vi "VI Scripting with Structures - Event Structure.vi"   [LabVIEW 2019]
doc: "This example contains sample code demonstrating common VI Scripting navigational tasks relating to Event Structures."
uses:
  <vilib>/Utility/traverseref.llb/TRef TravTarget.ctl
  <vilib>/event_ctls.llb/lveventtype.ctl
  <vilib>/Utility/traverseref.llb/VI Scripting - Traverse.lvlib
panel:
  # "Overview: Illustrates several EventStructure properties and methods used for inspecting and modifying Event Structures with VI Scripting.\nInstructions:\nOpen the block diagram of this VI to see several examples of properties and methods related to Event Structures and VI Scripting.\n\nNote: Browse the diagram of this example to learn about VI Scripting concepts. This example is not meant to be run."
types:
  T1 = typedef "lveventtype.ctl" = enum32{"Null", "Timeout", "Annotation Menu Selection", "Annotation Menu Selection?", "App Instance Close", "App Instance Close?", "Autoscale Range Change", "Bookmark Info Change", "Cell Edit", "Cell Edit?", "Cursor Grab", "Cursor Grab?", "Cursor Menu Selection", "Cursor Menu Selection?", "Cursor Move", "Cursor Release", "Data Change", "Direction Change", "Display State Change", "Drag Ended", "Drag Enter", "Drag Leave", "Drag Over", "Drag Source Update", "Drag Starting", "Drag Starting?", "Drop", "Exec State Change", "Key Down", "Key Down?", "Key Repeat", "Key Repeat?", "Key Up", "Listbox Double Click", "Menu Activation?", "Menu Selection (App)", "Menu Selection? (App)", "Menu Selection (User)", "Mouse Down", "Mouse Down?", "Mouse Enter", "Mouse Leave", "Mouse Move", "Mouse Up", "Mouse Wheel", "NI Security User Change (App)", "Pane Size", "Panel Close", "Panel Close?", "Panel Resize", "Plot Attribute Change", "Scale Range Change", "Shortcut Menu Activation?", "Shortcut Menu Selection (App)", "Shortcut Menu Selection? (App)", "Shortcut Menu Selection (User)", "Tree Double Click", "Tree Drag", "Tree Drag?", "Tree Drop", "Tree Drop?", "Tree Item Close", "Tree Item Close?", "Tree Item Open", "Tree Item Open?", "User Event", "Value Change"}
  T2 = cluster{"Event Type":T1, "Event Registration Index":i32}[]
  T3 = enum32{"Null", "Timeout", "Annotation Menu Selection", "Annotation Menu Selection?", "App Instance Close", "App Instance Close?", "Autoscale Range Change", "Bookmark Info Change", "Cell Edit", "Cell Edit?", "Cursor Grab", "Cursor Grab?", "Cursor Menu Selection", "Cursor Menu Selection?", "Cursor Move", "Cursor Release", "Data Change", "Direction Change", "Display State Change", "Drag Ended", "Drag Enter", "Drag Leave", "Drag Over", "Drag Source Update", "Drag Starting", "Drag Starting?", "Drop", "Exec State Change", "Key Down", "Key Down?", "Key Repeat", "Key Repeat?", "Key Up", "Listbox Double Click", "Menu Activation?", "Menu Selection (App)", "Menu Selection? (App)", "Menu Selection (User)", "Mouse Down", "Mouse Down?", "Mouse Enter", "Mouse Leave", "Mouse Move", "Mouse Up", "Mouse Wheel", "NI Security User Change (App)", "Pane Size", "Panel Close", "Panel Close?", "Panel Resize", "Plot Attribute Change", "Scale Range Change", "Shortcut Menu Activation?", "Shortcut Menu Selection (App)", "Shortcut Menu Selection? (App)", "Shortcut Menu Selection (User)", "Tree Double Click", "Tree Drag", "Tree Drag?", "Tree Drop", "Tree Drop?", "Tree Item Close", "Tree Item Close?", "Tree Item Open", "Tree Item Open?", "User Event", "Value Change"}
  T4 = cluster{"Event Type":T1, "Limit (-1=none)":i32, "Lock Panel?":bool}[]
  T5 = typedef "TRef TravTarget.ctl" = enum16{"FP", "BD", "Other"}
  T6 = cluster{"Event Type":enum32{"Null", "Timeout", "Annotation Menu Selection", "Annotation Menu Selection?", "App Instance Close", "App Instance Close?", "Autoscale Range Change", "Bookmark Info Change", "Cell Edit", "Cell Edit?", "Cursor Grab", "Cursor Grab?", "Cursor Menu Selection", "Cursor Menu Selection?", "Cursor Move", "Cursor Release", "Data Change", "Direction Change", "Display State Change", "Drag Ended", "Drag Enter", "Drag Leave", "Drag Over", "Drag Source Update", "Drag Starting", "Drag Starting?", "Drop", "Exec State Change", "Key Down", "Key Down?", "Key Repeat", "Key Repeat?", "Key Up", "Listbox Double Click", "Menu Activation?", "Menu Selection (App)", "Menu Selection? (App)", "Menu Selection (User)", "Mouse Down", "Mouse Down?", "Mouse Enter", "Mouse Leave", "Mouse Move", "Mouse Up", "Mouse Wheel", "NI Security User Change (App)", "Pane Size", "Panel Close", "Panel Close?", "Panel Resize", "Plot Attribute Change", "Scale Range Change", "Shortcut Menu Activation?", "Shortcut Menu Selection (App)", "Shortcut Menu Selection? (App)", "Shortcut Menu Selection (User)", "Tree Double Click", "Tree Drag", "Tree Drag?", "Tree Drop", "Tree Drop?", "Tree Item Close", "Tree Item Close?", "Tree Item Open", "Tree Item Open?", "User Event", "Value Change"}, "Reference":refnum<vi>, "Limit (-1=none)":i32, "Lock Panel?":bool}
  T7 = cluster{"Event Type":enum32{"Null", "Timeout", "Annotation Menu Selection", "Annotation Menu Selection?", "App Instance Close", "App Instance Close?", "Autoscale Range Change", "Bookmark Info Change", "Cell Edit", "Cell Edit?", "Cursor Grab", "Cursor Grab?", "Cursor Menu Selection", "Cursor Menu Selection?", "Cursor Move", "Cursor Release", "Data Change", "Direction Change", "Display State Change", "Drag Ended", "Drag Enter", "Drag Leave", "Drag Over", "Drag Source Update", "Drag Starting", "Drag Starting?", "Drop", "Exec State Change", "Key Down", "Key Down?", "Key Repeat", "Key Repeat?", "Key Up", "Listbox Double Click", "Menu Activation?", "Menu Selection (App)", "Menu Selection? (App)", "Menu Selection (User)", "Mouse Down", "Mouse Down?", "Mouse Enter", "Mouse Leave", "Mouse Move", "Mouse Up", "Mouse Wheel", "NI Security User Change (App)", "Pane Size", "Panel Close", "Panel Close?", "Panel Resize", "Plot Attribute Change", "Scale Range Change", "Shortcut Menu Activation?", "Shortcut Menu Selection (App)", "Shortcut Menu Selection? (App)", "Shortcut Menu Selection (User)", "Tree Double Click", "Tree Drag", "Tree Drag?", "Tree Drop", "Tree Drop?", "Tree Item Close", "Tree Item Close?", "Tree Item Open", "Tree Item Open?", "User Event", "Value Change"}, "Reference":refnum<vi>, "Limit (-1=none)":i32, "Lock Panel?":bool}[]
  T8 = cluster{"Event Type":T1, "Reference":refnum<vi>, "Limit (-1=none)":i32, "Lock Panel?":bool}[]
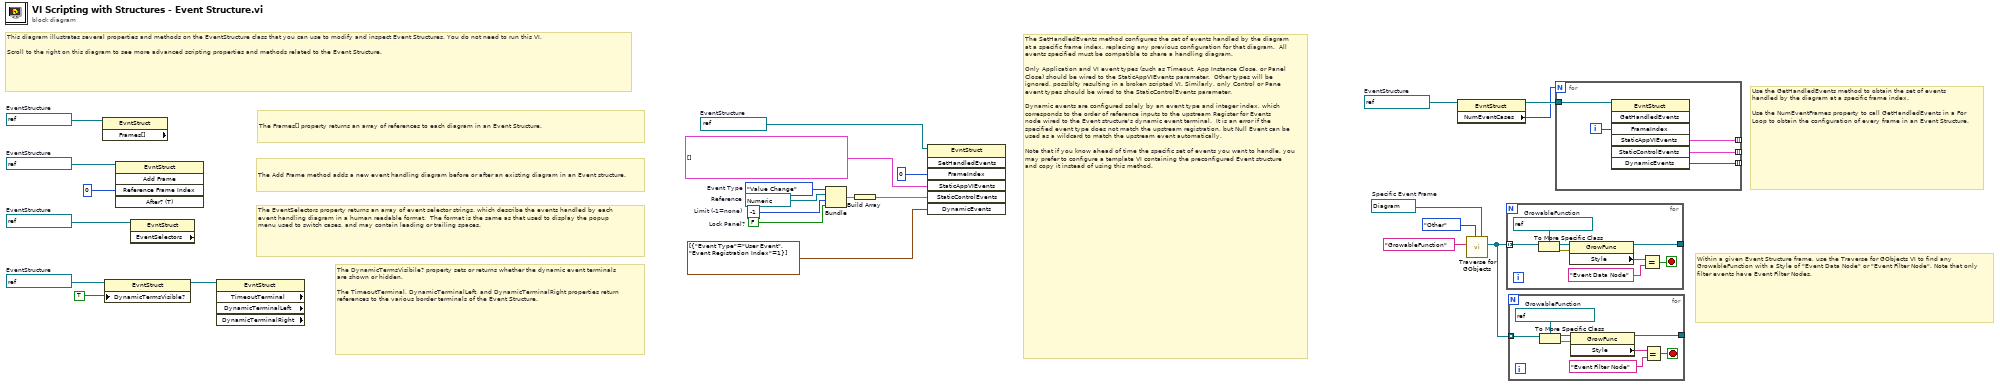
[diagram p0: block diagram]
diagram:
  w5 = refnum<vi> refnum  # EventStructure
  w6 = refnum<vi> refnum  # EventStructure
  w1 = refnum<vi> refnum  # EventStructure
  w10 = refnum<vi> refnum  # EventStructure
  w16 = refnum<vi> refnum  # Reference
  w14 = FALSE  # Lock Panel?
  w15 = -1  # Limit (-1=none)
  w17 = T3."Value Change"  # Event Type
  w11 = refnum<vi> refnum  # EventStructure
  w23 = refnum<vi> refnum  # Specific Event Frame
  w24 = refnum<vi> refnum  # EventStructure
  # "The DynamicTermsVisibile? property sets or returns whether the dynamic event terminals are shown or hidden.\n\nThe TimeoutTerminal, DynamicTerminalLeft, and DynamicTerminalRight properties return references to the various border terminals of the Event Structure."
  # "The EventSelectors property returns an array of event selector strings, which describe the events handled by each event handling diagram in a human readable format.  The format is the same as that used to display the popup menu used to switch cases, and may contain leading or trailing spaces."
  # "Use the GetHandledEvents method to obtain the set of events handled by the diagram at a specific frame index.\n\nUse the NumEventFrames property to call GetHandledEvents in a For Loop to obtain the configuration of every frame in an Event Structure."
  # "The SetHandledEvents method configures the set of events handled by the diagram at a specific frame index, replacing any previous configuration for that diagram.  All events specified must be compatible to share a handling diagram.\n\nOnly Application and VI event types (such as Timeout, App Instance Close, or Panel Close) should be wired to the StaticAppVIEvents parameter.  Other types will be ignored, possiblty resulting in a broken scripted VI. Similarly, only Control or Pane event types should be wired to the StaticControlEvents parameter.\n\nDynamic events are configured solely by an event type and integer index, which corresponds to the order of reference inputs to the upstream Register for Events node wired to the Event structure's dynamic event terminal.  It is an error if the specified event type does not match the upstream registration, but Null Event can be used as a wildcard to match the upstream event automatically.\n\nNote that if you know ahead of time the specific set of events you want to handle, you may prefer to configure a template VI containing the preconfigured Event structure and copy it instead of using this method."
  # "The Add Frame method adds a new event handling diagram before or after an existing diagram in an Event structure."
  # "The Frames[] property returns an array of references to each diagram in an Event Structure."
  # "This diagram illustrates several properties and methods on the EventStructure class that you can use to modify and inspect Event Structures. You do not need to run this VI.\n\nScroll to the right on this diagram to see more advanced scripting properties and methods related to the Event Structure."
  # "Within a given Event Structure frame, use the Traverse for GObjects VI to find any GrowableFunction with a Style of \"Event Data Node\" or \"Event Filter Node\". Note that only filter events have Event Filter Nodes."
  n1 = property class="EvntStruct" props=["Frames[]"](reference=w24) -> ()  [unwired: 1 in, 3 out]
  n2 = property class="EvntStruct"(reference=w6, "DynamicTermsVisible?"=TRUE ("Dynamic Terminals Visible?")) -> (reference out=w8:refnum<vi>)  [unwired: 1 in, 1 out]
  n3 = invoke class="EvntStruct" method="Add Frame"(reference=w11, "Reference Frame Index"=u32 0) -> ()  [unwired: 3 in, 5 out]
  n4 = property class="EvntStruct" props=["EventSelectors"](reference=w5) -> ()  [unwired: 1 in, 3 out]
  n5 = property class="EvntStruct" props=["TimeoutTerminal", "DynamicTerminalLeft", "DynamicTerminalRight"](reference=w8) -> ()  [unwired: 1 in, 5 out]
  n6 = Bundle("Event Type"=w17, "Reference"=w16, "Limit (-1=none)"=w15, "Lock Panel?"=w14) -> (w13:T6)  [unwired: 1 in]
  n7 = Build Array(w13) -> (w9:T7)
  n8 = invoke class="EvntStruct" method="SetHandledEvents"(reference=w10, "FrameIndex"=0 ("Frame Index"), "StaticAppVIEvents"=T4 [] ("Static App/VI Events"), "StaticControlEvents"=w9, "DynamicEvents"=T2 [{"Event Type"=enum."User Event", "Event Registration Index"=1}] ("Dynamic Events")) -> ()  [unwired: 2 in, 7 out]
  n9 = property class="EvntStruct"(reference=w1) -> (reference out=w3:refnum<vi>, "NumEventCases"=w2:i32)  [unwired: 1 in, 1 out]
  n10 = call <vilib>:"Traverse for GObjects.vi"("Other Refnum"=w23, "Traverse Target"=TRef_TravTarget."Other", "Class Name"="GrowableFunction") -> ("References"=w20:refnum<vi>[])  [unwired: 5 in, 3 out]
  n11 = for {
    tunnel: w20 -> [w32] mode=indexing
    tunnel: [w28] -> _
    stop <- w25 stop-if-true
    w31 = refnum<vi> refnum  # GrowableFunction
    n12 = To More Specific Class(target class=w31, reference=w32) -> (specific class reference=w30:refnum<vi>, error out=w29:errorcluster)  [unwired: 1 in]
    n13 = property class="GrowFunc"(reference=w30, error in=w29) -> (reference out=w28:refnum<vi>, "Style"=w27:string)  [unwired: 1 out]
    n14 = Equal?(x=w27, y="Event Data Node" ("Style")) -> (x = y?=w25:bool)
  }
  n15 = for {
    tunnel: w20 -> [w40] mode=indexing
    tunnel: [w36] -> _
    stop <- w33 stop-if-true
    w39 = refnum<vi> refnum  # GrowableFunction
    n16 = To More Specific Class(target class=w39, reference=w40) -> (specific class reference=w38:refnum<vi>, error out=w37:errorcluster)  [unwired: 1 in]
    n17 = property class="GrowFunc"(reference=w38, error in=w37) -> (reference out=w36:refnum<vi>, "Style"=w35:string)  [unwired: 1 out]
    n18 = Equal?(x=w35, y="Event Filter Node" ("Style")) -> (x = y?=w33:bool)
  }
  n19 = for {
    N: w2 -> [_]
    tunnel: w3 -> [w45]
    tunnel: [w44] -> _ mode=indexing
    tunnel: [w43] -> _ mode=indexing
    tunnel: [w42] -> _ mode=indexing
    i -> [w41]
    n20 = invoke class="EvntStruct" method="GetHandledEvents"(reference=w45, "FrameIndex"=w41) -> ("StaticAppVIEvents"=w44:T4, "StaticControlEvents"=w43:T8, "DynamicEvents"=w42:T2)  [unwired: 5 in, 4 out]
  }
